vi "PYTHON Set Integer Matrix__ogtk.vi"(4 "error in (no error)":errorcluster, 5 "value":i32[][](array[numeric]), 6 "variable name":string, 7 "Python Session in":T1) -> (0 "error out":errorcluster, 3 "Python Session out":T1)   [LabVIEW 2014]
uses:
  <userlib>/_OpenG.lib/labpython/labpython.llb/PYTHON Session Refnum__ogtk.ctl
  <userlib>/_OpenG.lib/labpython/lvpython.dll
panel:
  # "PYTHON Set Integer Matrix.vi\n\nSet the value of an integer matrix variable in the session context\n\nCopyright (C) 2002 Rolf Kalbermatter rolf.kalbermatter@citeng.com\nCopyright (C) 2002 James Kring jim@jimkring.com\n\nPlease visit http://www.OpenG.org to learn about the\nOpen Source LabVIEW software movement.\n\nThis library is free software; you can redistribute it and/or\nmodify it under the terms of the GNU Lesser General Public\nLicense as published by the Free Software Foundation; either\nversion 2.1 of the License, or (at your option) any later version.\nThis library is distributed in the hope that it will be useful,\nbut WITHOUT ANY WARRANTY; without even the implied warranty of\nMERCHANTABILITY or FITNESS FOR A PARTICULAR PURPOSE. See the GNU\nLesser General Public License for more details.\nYou should have received a copy of the GNU Lesser General Public\nLicense along with this library; if not, write to the Free Software\nFoundation, Inc., 59 Temple Place, Suite 330, Boston, MA 02111-1307 USA"
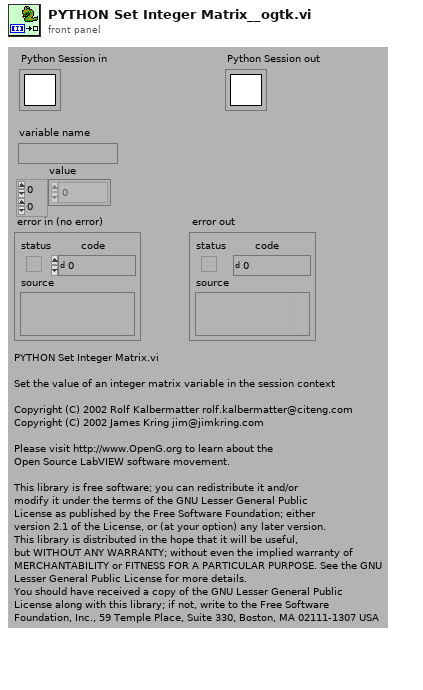
[diagram p1: front panel]
types:
  T1 = typedef "PYTHON Session Refnum__ogtk.ctl" = refnum<k1>
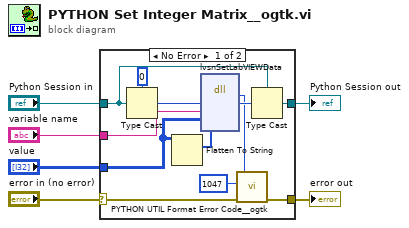
[diagram p0: block diagram]
diagram:
  n1 = case shown="No Error" "error in (no error)" {
    selector: "error in (no error)" -> [w15 w20]
    tunnel: [w13 w20] -> w5
    tunnel: "variable name" -> [w18 _]
    tunnel: "value" -> [w12 _]
    tunnel: "Python Session in" -> [w8 w19]
    tunnel: [w7 w19] -> w1
    frame No Error {
      n2 = Type Cast(type=u32 0 ("session"), x=w8) -> (*(type *) &x=w9:u32)
      n3 = Flatten To String(anything=w12) -> (type string=w11:i16[])  [unwired: 3 in, 2 out]
      n4 = dll-call lib="C:/Program Files (x86)/National Instruments/LabVIEW 2014/user.lib/_OpenG.lib/labpython/lvpython.*" fn="lvsnSetLabVIEWData"("session"=w9, "name"=w18, "value"=w12, "type"=w11) -> (w14:i32, "session"=w17:u32)  [unwired: 6 in, 2 out]
      n5 = call <userlib>:"PYTHON UTIL Format Error Code__ogtk.vi"("error in (no error)"=w15, "code"=1047, "Bool32"=w14) -> ("error out"=w13:errorcluster)  [unwired: 4 in]
      n6 = Type Cast(type=w8, x=w17) -> (*(type *) &x=w7:T1)
    }
    frame Error {
    }
  }
  "error out" <- w5
  "Python Session out" <- w1
